vi "choose_state.vi"(6 "v2":dbl, 7 "v1":dbl, 8 "d2":dbl, 9 "d1":dbl, 10 "from_right2":i16, 11 "from_right1":i16) -> (2 "state":i16)   [LabVIEW 2022 SP3]
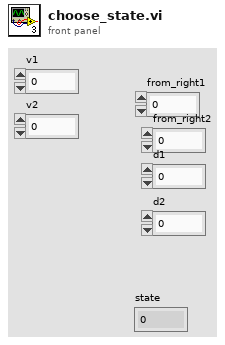
[diagram p1: front panel]
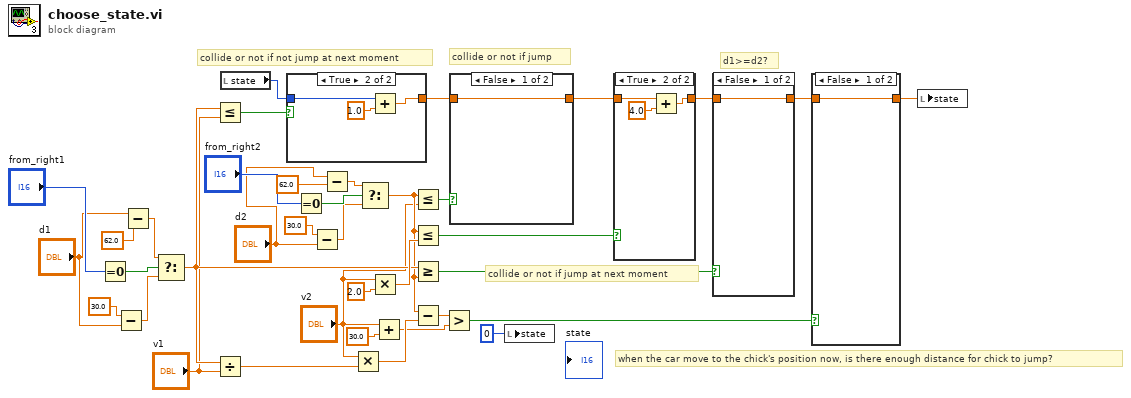
[diagram p0: block diagram]
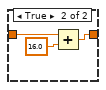
[diagram p2: hidden frame]
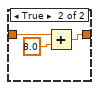
[diagram p3: hidden frame]
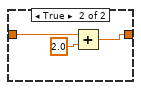
[diagram p5: hidden frame]
diagram:
  # "when the car move to the chick's position now, is there enough distance for chick to jump?"
  # "d1>=d2?"
  # "collide or not if jump at next moment"
  # "collide or not if not jump at next moment"
  # "collide or not if jump"
  # "collide or not if not jump at next moment"
  n1 = Equal To 0?(x="from_right1") -> (x = 0?=w34:bool)
  n2 = Subtract(x=30.0, y="d1") -> (x-y=w32:dbl)
  n3 = Subtract(x="d1", y=62.0 ("x")) -> (x-y=w6:dbl)
  n4 = Select(t=w6, s=w34, f=w32) -> (s? t:f=w22:dbl)
  n5 = Less Or Equal?(x=w22, y="v1") -> (x <= y?=w29:bool)
  n6 = Divide(x=w22, y="v1") -> (x/y=w20:dbl)
  n7 = local read "state"() -> (w23:i16)
  n8 = case shown="True" w29 {
    tunnel: w23 -> [w38 w40]
    tunnel: [w38 w39] -> w11
    frame False {
    }
    frame True {
      n9 = Add(x=w40, y=1.0) -> (x+y=w39:dbl)
    }
  }
  n10 = Equal To 0?(x="from_right2") -> (x = 0?=w35:bool)
  n11 = Subtract(x=30.0, y="d2") -> (x-y=w30:dbl)
  n12 = Subtract(x="d2", y=62.0 ("x")) -> (x-y=w1:dbl)
  n13 = Multiply(x="v2", y=w20) -> (x*y=w19:dbl)
  n14 = Select(t=w1, s=w35, f=w30) -> (s? t:f=w18:dbl)
  n15 = Multiply(x="v2", y=2.0) -> (x*y=w26:dbl)
  n16 = Add(x="v2", y=30.0) -> (x+y=w16:dbl)
  n17 = Less Or Equal?(x=w18, y="v2") -> (x <= y?=w27:bool)
  n18 = Less Or Equal?(x=w18, y=w26) -> (x <= y?=w12:bool)
  n19 = Greater Or Equal?(x=w22, y=w18) -> (x >= y?=w24:bool)
  n20 = Subtract(x=w18, y=w19) -> (x-y=w17:dbl)
  n21 = Greater?(x=w17, y=w16) -> (0:w13:bool)
  n22 = case shown="False" w27 {
    tunnel: w11 -> [w42 w44]
    tunnel: [w42 w43] -> w10
    frame False {
    }
    frame True {
      n23 = Add(x=w44, y=2.0) -> (x+y=w43:dbl)
    }
  }
  n24 = local write "state"(i16 0 ("state")) -> ()
  n25 = case shown="True" w12 {
    tunnel: w10 -> [w46 w48]
    tunnel: [w46 w47] -> w9
    frame False {
    }
    frame True {
      n26 = Add(x=w48, y=4.0) -> (x+y=w47:dbl)
    }
  }
  n27 = case shown="False" w24 {
    tunnel: w9 -> [w50 w52]
    tunnel: [w50 w51] -> w8
    frame False {
    }
    frame True {
      n28 = Add(x=w52, y=8.0) -> (x+y=w51:dbl)
    }
  }
  n29 = case shown="False" w13 {
    tunnel: w8 -> [w54 w56]
    tunnel: [w54 w55] -> w7
    frame False {
    }
    frame True {
      n30 = Add(x=w56, y=16.0) -> (x+y=w55:dbl)
    }
  }
  n31 = local write "state"(w7) -> ()
